vi "ZCR - remove transients.vi"(6 "State":enum16{"ON", "OFF"}(ring), 8 "(i)":i32, 9 "lim d(f)":dbl=200.0, 10 "d(f)":dbl[](array[numeric]), 11 "delta":dbl) -> (3 "OK ?":bool)   [LabVIEW 2020, in "Library Commun.lvlib" / "Nodon_ZCR.lvclass"]
uses:
  Nodon_ZCR.lvclass
  Nodon_ZCR.lvclass/Nodon_ZCR.ctl
panel:
  # "This VI prevents small transients signals to be mistaken for front detection\nusing the derivative analysis method"
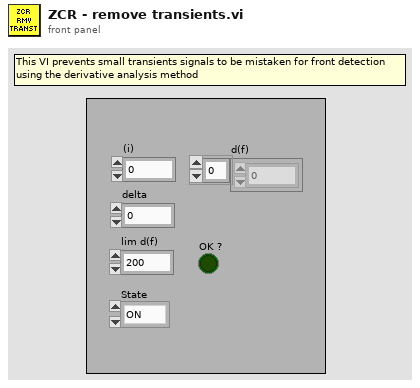
[diagram p1: front panel]
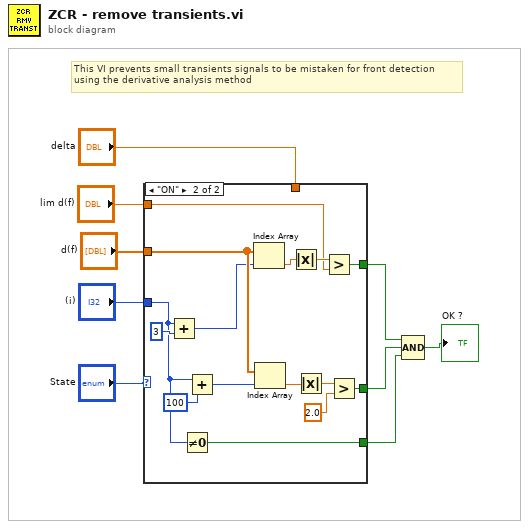
[diagram p0: block diagram]
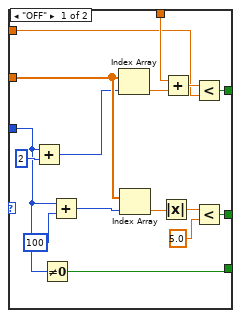
[diagram p2: hidden frame]
diagram:
  # "This VI prevents small transients signals to be mistaken for front detection\nusing the derivative analysis method"
  n1 = case shown="\"ON\"" "State" {
    tunnel: "delta" -> [w23 _]
    tunnel: "lim d(f)" -> [w22 w29]
    tunnel: "d(f)" -> [w20 w39]
    tunnel: [w16 w31] -> w6
    tunnel: [w15 w35] -> w5
    tunnel: "(i)" -> [w10 w27]
    tunnel: [w11 w26] -> w1
    frame "OFF" {
      n2 = Add(x=w10, y=2) -> (x+y=w14:i32)
      n3 = Not Equal To 0?(x=w10) -> (x != 0?=w11:bool)
      n4 = Add(x=w10, y=100) -> (x+y=w21:i32)
      n5 = Index Array(array=w20, index=w14) -> (element=w25:dbl)
      n6 = Index Array(array=w20, index=w21) -> (element=w19:dbl)
      n7 = Absolute Value(x=w19) -> (abs(x)=w18:dbl)
      n8 = Add(x=w23, y=w25) -> (x+y=w24:dbl)
      n9 = Less?(x=w24, y=w22) -> (x < y?=w16:bool)
      n10 = Less?(x=w18, y=5.0) -> (x < y?=w15:bool)
    }
    frame "ON" {
      n11 = Add(x=w27, y=3) -> (x+y=w34:i32)
      n12 = Not Equal To 0?(x=w27) -> (x != 0?=w26:bool)
      n13 = Add(x=w27, y=100) -> (x+y=w40:i32)
      n14 = Index Array(array=w39, index=w34) -> (element=w30:dbl)
      n15 = Index Array(array=w39, index=w40) -> (element=w38:dbl)
      n16 = Absolute Value(x=w30) -> (abs(x)=w32:dbl)
      n17 = Absolute Value(x=w38) -> (abs(x)=w37:dbl)
      n18 = Greater?(x=w32, y=w29) -> (0:w31:bool)
      n19 = Greater?(x=w37, y=2.0) -> (0:w35:bool)
    }
  }
  n20 = Compound Arithmetic op=AND(w6, w5, w1) -> (→"OK ?":bool)
